vi "Get Communication Profile Objects.vi"(8 "error in":errorcluster, 11 "Obj Dict in":refnum<class "Object Dictionary.lvclass">) -> (0 "error out":errorcluster, 2 "Communcation Profile":refnum<class "Object Entry.lvclass">[](array[class]), 3 "Obj Dict out":refnum<class "Object Dictionary.lvclass">)   [LabVIEW 2020, in "CANopen.lvlib" / "Object Dictionary.lvclass"]
uses:
  Object Dictionary.lvclass
  Object Entry/Object Entry.lvclass
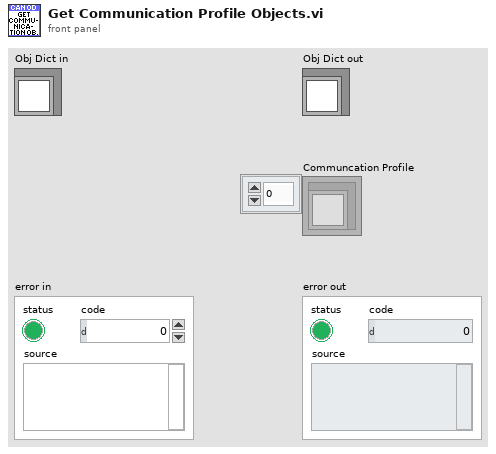
[diagram p1: front panel]
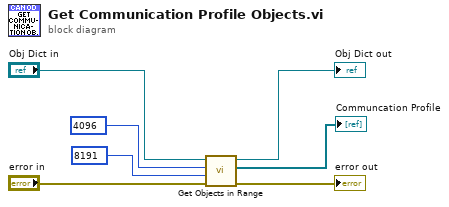
[diagram p0: block diagram]
diagram:
  n1 = call "Get Objects in Range.vi"("error in"="error in", "End"=u16 8191, "Start"=u16 4096, "Obj Dict in"="Obj Dict in") -> ("error out"=→"error out":errorcluster, "Objects in Range"=→"Communcation Profile":refnum<class "Object Entry.lvclass">[], "Obj Dict out"=→"Obj Dict out":refnum<class "Object Dictionary.lvclass">)  [unwired: 5 in]
